vi "DFD MRate Filter Design (Integer).vi"(4 "filtering mode":T9=2 items=["No Rate Change", "Interpolation", "Decimation"], 5 "method":u16(ring)=2 items=["Kaiser Window", "Dolph-Chebyshev Window", "Equi-Ripple"], 6 "fs in [Hz]":dbl=800.0, 7 "factor":i32=8, 8 "error in (no error)":errorcluster, 9 "ripple specs":T2={"passband"=0.1, "stopband"=60.0, "dB/linear? (T: dB)"=TRUE}, 10 "freq specs [Hz]":T3={"fpass"=45.0, "fstop"=52.0}, 11 "order":i32=-1) -> (0 "error out":errorcluster, 3 "multirate filter out":T4={"mMRate_Structure"=enum."IIR", "mMRate_Mode"=0, "mMRate_Factor"=-1, "mMRate_FIRParams"={"mMRate_FIR_H"=[], "mMRate_FIR_IsNyquist?"=FALSE, "mMRate_FIR_IsSymmetric?"=FALSE}, "mMRate_CICParams"={"mMRate_CIC_#Stage"=0, "mMRate_CIC_Lag"=0, "mMRate_CIC_Type"=enum."Lowpass"}, "mMRate_Order"=0, "mMRate_Version"="2.0", "mMRate_Comments"="", "mMRate_RationalFactor"={"mMRate_L"=-1, "mMRate_M"=-1}, "mMRate_Fs"=1.0, "mMRate_Quantized?"=FALSE, "mMRate_QFilterGain"=1.0, "mMRate_CoefWl"=16, "mMRate_Scaling"={"mMRate_ScaleByPowerOf2?"=FALSE, "mMRate_ScaleType"=enum."No Norm"}, "mMRate_InputWl"=16, "mMRate_OutputWl"=16, "mMRate_OutputMode"=enum."Truncation", "mMRate_MultMode"=enum."Truncated", "mMRate_BitPruning"=FALSE, "mMRate_GainWl"=16, "mMRate_OutputFwl"=0, "mMRate_SumIwl"=0, "mMRate_InputIwl "=16, "mMRate_SumWl"=32, "mMRate_CoefIwl"=0} {"mMRate_SumWl" min=1 max=32 step=1; "mMRate_InputIwl" min=1 max=32 step=1; "mMRate_GainWl" min=1 max=32 step=1; "mMRate_OutputWl" min=1 max=32 step=1; "mMRate_InputWl" min=1 max=32 step=1; "mMRate_CoefWl" min=1 max=32 step=1; "mMRate_Mode" items=["Default"=-1, "No Rate Change"=0, "Interpolation"=1, "Decimation"=2, "Interpolated"=3, "Rational"=4]})   [LabVIEW 2017, in "NI_DigFilterLicensed.lvlib"]
doc: "Creates a single-stage multirate filter. You must manually select the polymorphic instance you want to use."
uses:
  <vilib>/addons/Digital Filter Design/NI_DigFilterLicensed.lvlib
  <vilib>/addons/Digital Filter Design/_Objects.llb/DFD Multirate Filtering Mode.ctl
  <vilib>/addons/Digital Filter Design/_Objects.llb/DFD Multirate Filter Obj.ctl
  <vilib>/addons/Digital Filter Design/_Objects.llb/DFD Multirate Mode.ctl
  <vilib>/addons/Digital Filter Design/_Objects.llb/DFD Coef Norm Type.ctl
  <vilib>/addons/Digital Filter Design/_Objects.llb/DFD Round-off Mode.ctl
  <vilib>/addons/Digital Filter Design/_Objects.llb/DFD FXP MRate Multiply Mode.ctl
  <vilib>/addons/Digital Filter Design/_Objects.llb/DFD Multirate Filter Specification (Design).ctl
  <vilib>/addons/Digital Filter Design/_Objects.llb/DFD Filter Ripple Specification (Design).ctl
  <vilib>/addons/Digital Filter Design/_Objects.llb/DFD Adv Band Spec.ctl
  <vilib>/addons/Digital Filter Design/FilterLib.llb/DFD Build MRate Filter from FIR Filter.vi
  <vilib>/addons/Digital Filter Design/NI_DigFilter_Process.lvlib
  <vilib>/addons/Digital Filter Design/NI_DigFilter_Design.lvlib
panel:
  in  "band 2":T1
  # "freq"
  # "amplitude"
  # "weight"
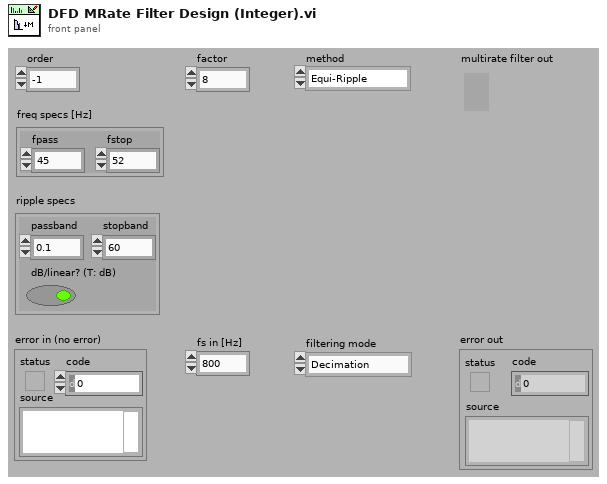
[diagram p1: front panel]
types:
  T1 = typedef "NI_DigFilterLicensed.lvlib/DFD Adv Band Spec.ctl" = cluster{"band specification":cluster{"freq":dbl, "amplitude":dbl, "weight":dbl}[], "ripple constraint":dbl}
  T2 = typedef "NI_DigFilterLicensed.lvlib/DFD Filter Ripple Specification (Design).ctl" = cluster{"passband":dbl, "stopband":dbl, "dB/linear? (T: dB)":bool}
  T3 = typedef "NI_DigFilterLicensed.lvlib/DFD Multirate Filter Specification (Design).ctl" = cluster{"fpass":dbl, "fstop":dbl}
  T4 = typedef "NI_DigFilterLicensed.lvlib/DFD Multirate Filter Obj.ctl" = cluster{"mMRate_Structure":enum16{"CIC", "FIR", "IIR", "Lattice"}, "mMRate_Mode":T5, "mMRate_Factor":i32, "mMRate_FIRParams":cluster{"mMRate_FIR_H":dbl[], "mMRate_FIR_IsNyquist?":bool, "mMRate_FIR_IsSymmetric?":bool}, "mMRate_CICParams":cluster{"mMRate_CIC_#Stage":i32, "mMRate_CIC_Lag":i32, "mMRate_CIC_Type":enum16{"Lowpass", "Highpass"}}, "mMRate_Order":i32, "mMRate_Version":string, "mMRate_Comments":string, "mMRate_RationalFactor":cluster{"mMRate_L":i32, "mMRate_M":i32}, "mMRate_Fs":dbl, "mMRate_Quantized?":bool, "mMRate_QFilterGain":dbl, "mMRate_CoefWl":i16, "mMRate_Scaling":cluster{"mMRate_ScaleByPowerOf2?":bool, "mMRate_ScaleType":T6}, "mMRate_InputWl":i16, "mMRate_OutputWl":i16, "mMRate_OutputMode":T7, "mMRate_MultMode":T8, "mMRate_BitPruning":bool, "mMRate_GainWl":i16, "mMRate_OutputFwl":i16, "mMRate_SumIwl":i16, "mMRate_InputIwl ":i16, "mMRate_SumWl":i16, "mMRate_CoefIwl":i16}
  T5 = typedef "NI_DigFilterLicensed.lvlib/DFD Multirate Mode.ctl" = i16
  T6 = typedef "NI_DigFilterLicensed.lvlib/DFD Coef Norm Type.ctl" = enum16{"No Norm", "Time Domain 1-Norm", "Time Domain 2-Norm", "Time Domain Inf-Norm"}
  T7 = typedef "NI_DigFilterLicensed.lvlib/DFD Round-off Mode.ctl" = enum16{"Nearest", "Truncation"}
  T8 = typedef "NI_DigFilterLicensed.lvlib/DFD FXP MRate Multiply Mode.ctl" = enum16{"Truncated", "Full"}
  T9 = typedef "NI_DigFilterLicensed.lvlib/DFD Multirate Filtering Mode.ctl" = u16
  T10 = enum16{"Butterworth", "Chebyshev", "Inverse Chebyshev", "Elliptic", "Kaiser Window", "Dolph-Chebyshev Window", "Equi-Ripple FIR"}
  T11 = typedef "NI_DigFilterLicensed.lvlib/DFD Filter Obj.ctl" = cluster{"mSRate_Fs":dbl, "mSRate_Version":string, "mSRate_Comments":string, "mSRate_OrgCoef":T12, "mSRate_CurCoef":T12, "mSRate_Quantized?":bool, "mSRate_QCoef":T12, "mSRate_QSettings":T14[], "mSRate_Order":i32, "mSRate_Scaling":cluster{"mSRate_ScaleByPowerOf2?":bool, "mSRate_ScaleType":T6}}
  T12 = typedef "NI_DigFilterLicensed.lvlib/DFD Filter Coef.ctl" = cluster{"type":T13, "gain":dbl, "coef a (k)":dbl[], "coef b (v)":dbl[]}
  T13 = typedef "NI_DigFilterLicensed.lvlib/DFD Filter Structure Type Selector.ctl" = enum16{"Undefined", "FIR Direct Form", "FIR Direct Form Transposed", "FIR Symmetric", "FIR Antisymmetric", "IIR Direct Form I", "IIR Direct Form I Transposed", "IIR Direct Form II", "IIR Direct Form II Transposed", "IIR Cascaded Second Order Sections Form I", "IIR Cascaded Second Order Sections Form I Transposed", "IIR Cascaded Second Order Sections Form II", "IIR Cascaded Second Order Sections Form II Transposed", "Lattice Allpass (basic sections)", "Lattice Allpass (one multiplier sections)", "Lattice Allpass (normalized sections)", "Lattice AR (basic sections)", "Lattice AR (one multiplier sections)", "Lattice AR (normalized sections)", "Lattice MA (minimum phase)", "Lattice MA (maximum phase)", "Lattice ARMA (basic sections)", "Lattice ARMA (one multiplier sections)", "Lattice ARMA (normalized sections)"}
  T14 = typedef "NI_DigFilterLicensed.lvlib/dfd_Internal Quantization Settings.ctl" = cluster{"source":T15, "wl":i16, "iwl":i16, "overflow mode":enum16{"Saturation", "Wrap"}, "rounding mode":enum16{"Nearest", "Truncation"}, "signed?":bool}
  T15 = typedef "NI_DigFilterLicensed.lvlib/dfd_Internal Quantization Srcs.ctl" = u16
  T16 = cluster{"fpass":dbl, "fstop":dbl, "fstop":dbl, "fstop":dbl}
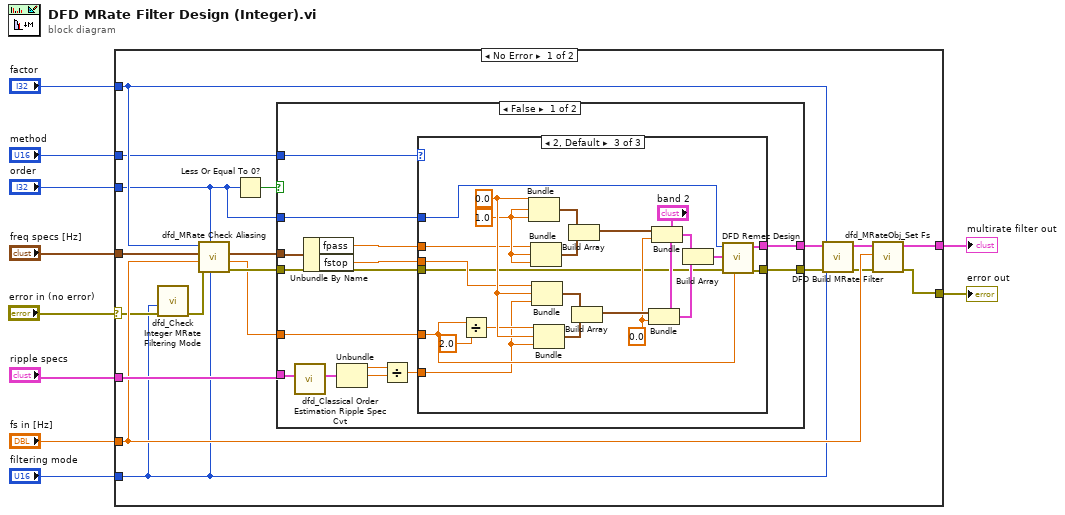
[diagram p0: block diagram]
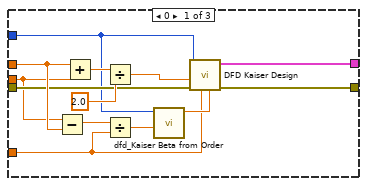
[diagram p2: hidden frame]
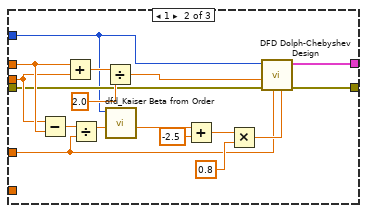
[diagram p3: hidden frame]
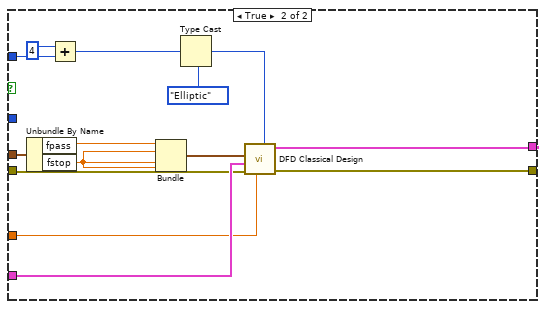
[diagram p4: hidden frame]
diagram:
  n1 = case shown="No Error" "error in (no error)" {
    selector: "error in (no error)" -> [w14 w110]
    tunnel: "freq specs [Hz]" -> [w28 _]
    tunnel: "fs in [Hz]" -> [w18 _]
    tunnel: "factor" -> [w23 _]
    tunnel: [w17 w110] -> w7
    tunnel: "order" -> [w20 _]
    tunnel: "ripple specs" -> [w24 _]
    tunnel: "method" -> [w21 _]
    tunnel: "filtering mode" -> [w12 _]
    tunnel: [w19 _] -> w2
    frame No Error {
      n2 = call <vilib>:"dfd_Check Integer MRate Filtering Mode.vi"("error IO"=w14, "filtering mode"=w12) -> ("error out"=w13:errorcluster)  [unwired: 9 out]
      n3 = call <vilib>:"dfd_MRate Check Aliasing.vi"("filtering mode"=w12, "order"=w20, "error in"=w13, "fs in [Hz]"=w18, "freq specs"=w28, "factor"=w23) -> ("error out"=w25:errorcluster, "filter fs [Hz]"=w11:dbl, "dup freq specs"=w26:T3)  [unwired: 3 out]
      n4 = Less Or Equal To 0?(x=w20) -> (x <= 0?=w27:bool)
      n5 = case shown="False" w27 {
        tunnel: w26 -> [w36 w99]
        tunnel: w25 -> [w39 w108]
        tunnel: w24 -> [w33 w109]
        tunnel: w21 -> [w42 w107]
        tunnel: w11 -> [w40 w104]
        tunnel: [w37 w103] -> w16
        tunnel: [w38 w102] -> w15
        tunnel: w20 -> [w41 _]
        frame False {
          n6 = call <vilib>:"dfd_Classical Order Estimation Ripple Spec Cvt.vi"("ripple specs"=w33) -> ("ripple specs (linear)"=w32:T2)  [unwired: 10 out]
          n7 = Unbundle By Name(w36) -> ("fpass"=w35:dbl, "fstop"=w34:dbl)
          n8 = Unbundle(w32) -> ("passband"=w31:dbl, "stopband"=w30:dbl)  [unwired: 1 out]
          n9 = Divide(x=w31, y=w30) -> (x/y=w29:dbl)
          n10 = case shown="2, Default" w42 {
            tunnel: [w47 w64 w78] -> w37
            tunnel: w35 -> [w53 w70 w84]
            tunnel: w34 -> [w43 w69 w83]
            tunnel: w41 -> [w49 w66 w79]
            tunnel: w40 -> [w44 w56 w76]
            tunnel: w39 -> [w50 w67 w80]
            tunnel: [w48 w65 w77] -> w38
            tunnel: w29 -> [_ _ w73]
            frame 0 {
              n11 = Subtract(x=w43, y=w53) -> (x-y=w45:dbl)
              n12 = Add(x=w53, y=w43) -> (x+y=w54:dbl)
              n13 = Divide(x=w54, y=2.0) -> (x/y=w52:dbl)
              n14 = Divide(x=w45, y=w44) -> (x/y=w46:dbl)
              n15 = call <vilib>:"dfd_Kaiser Beta from Order.vi"("delta f [Hz]"=w46, "order"=w49) -> ("beta"=w51:dbl)  [unwired: 9 out]
              n16 = call <vilib>:"DFD Kaiser Design.vi"("beta"=w51, "fs [Hz]"=w44, "error in (no error)"=w50, "low cutoff freq [Hz]"=w52, "order"=w49) -> ("error out"=w48:errorcluster, "filter out"=w47:T11)  [unwired: 2 in, 3 out]
            }
            frame 1 {
              n17 = Subtract(x=w69, y=w70) -> (x-y=w57:dbl)
              n18 = Add(x=w70, y=w69) -> (x+y=w71:dbl)
              n19 = Divide(x=w57, y=w56) -> (x/y=w58:dbl)
              n20 = Divide(x=w71, y=2.0) -> (x/y=w68:dbl)
              n21 = call <vilib>:"dfd_Kaiser Beta from Order.vi"("delta f [Hz]"=w58, "order"=w66) -> ("r [dB]"=w60:dbl)  [unwired: 9 out]
              n22 = Add(x=w60, y=-2.5) -> (x+y=w63:dbl)
              n23 = Multiply(x=w63, y=0.8) -> (x*y=w59:dbl)
              n24 = call <vilib>:"DFD Dolph-Chebyshev Design.vi"("ripple ratio [dB]"=w59, "fs [Hz]"=w56, "error in (no error)"=w67, "low cutoff freq [Hz]"=w68, "order"=w66) -> ("error out"=w65:errorcluster, "filter out"=w64:T11)  [unwired: 2 in, 3 out]
            }
            frame 2, Default {
              w85 = 0.0
              w86 = 1.0
              w88 = 0.0
              n25 = Divide(x=w76, y=2.0) -> (x/y=w74:dbl)
              n26 = Bundle(w88, w86, w86) -> (w95:cluster{dbl, dbl, dbl})  [unwired: 1 out]
              n27 = Bundle("fpass"=w84, w86, w86) -> (w94:cluster{"fpass":dbl, dbl, dbl})  [unwired: 1 out]
              n28 = Bundle("fstop"=w83, w88, w73) -> (w90:cluster{"fstop":dbl, dbl, dbl})  [unwired: 1 out]
              n29 = Bundle(w74, w88, w73) -> (w91:cluster{dbl, dbl, dbl})  [unwired: 1 out]
              n30 = Build Array(w95, w94) -> (w93:cluster{"fpass":dbl, dbl, dbl}[])
              n31 = Build Array(w90, w91) -> (w92:cluster{"fstop":dbl, dbl, dbl}[])
              n32 = Bundle(cluster="band 2", "band specification"=w92, "ripple constraint"=w85) -> (w89:T1)
              n33 = Bundle(cluster="band 2", "band specification"=w93, "ripple constraint"=w85) -> (w87:T1)
              n34 = Build Array(w87, w89) -> (w81:T1[])
              n35 = call <vilib>:"DFD Remez Design.vi"("fs [Hz]"=w76, "error in (no error)"=w80, "band specs"=w81, "order"=w79) -> ("error out"=w77:errorcluster, "filter out"=w78:T11)  [unwired: 3 in, 3 out]
            }
          }
        }
        frame True {
          n36 = Unbundle By Name(w99) -> ("fpass"=w98:dbl, "fstop"=w97:dbl)
          n37 = Add(x=u16 4, y=w107) -> (x+y=w101:u16)
          n38 = Bundle("fpass"=w98, "fstop"=w97, "fstop"=w97, "fstop"=w97) -> (w96:T16)  [unwired: 1 out]
          n39 = Type Cast(type=T10."Elliptic" ("design method"), x=w101) -> (*(type *) &x=w105:T10)
          n40 = call <vilib>:"DFD Classical Design.vi"("design method"=w105, "fs [Hz]"=w104, "error in (no error)"=w108, "ripple specs"=w109, "freq specs [Hz]"=w96) -> ("error out"=w102:errorcluster, "filter out"=w103:T11)  [unwired: 1 in, 4 out]
        }
      }
      n41 = call-poly <vilib>:"DFD Build MRate Filter.vi"("error in (no error)"=w15, "filtering mode"=w12, "factor"=w23, "filter in"=w16) -> ("error out"=w17:errorcluster, "multirate filter out"=w22:T4)  [unwired: 1 in, 5 out]
      n42 = call <vilib>:"dfd_MRateObj_Set Fs.vi"("fs"=w18, "multirate filter in"=w22) -> ("dup multirate filter"=w19:T4)  [unwired: 9 out]
    }
    frame Error {
    }
  }
  "multirate filter out" <- w2
  "error out" <- w7
